vi "getCalibrationLabels.vi"() -> (1 "size(s)":i32, 3 "filenames":string[](array[string]))   [LabVIEW 2022 SP3]
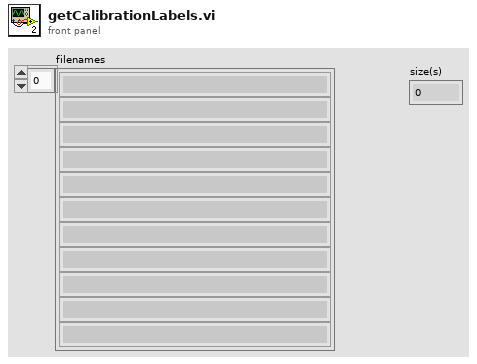
[diagram p1: front panel]
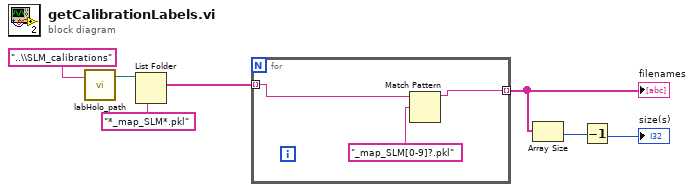
[diagram p0: block diagram]
diagram:
  n1 = call "labHolo_path.vi"("sub folder or file (str)"="..\\SLM_calibrations") -> ("labHolo path"=w4:path)  [unwired: 1 in, 1 out]
  n2 = List Folder(path=w4, pattern="*_map_SLM*.pkl") -> (filenames=w5:string[])  [unwired: 2 in, 3 out]
  n3 = for {
    tunnel: w5 -> [w8] mode=indexing
    tunnel: [w9] -> w3 mode=indexing
    n4 = Match Pattern(string=w8, regular expression="_map_SLM[0-9]?.pkl") -> (before substring=w9:string)  [unwired: 1 in, 3 out]
  }
  "filenames" <- w3
  n5 = Array Size(array=w3) -> (size(s)=w1:i32)
  n6 = Decrement(x=w1) -> (x-1=→"size(s)":i32)
